vi "Simple Client.vi"() -> ()   [LabVIEW 2023, in "Generated_client.lvlib"]
uses:
  Generated_client.lvlib
  RPC Messages/streamai_signalConfig.ctl
  RPC Messages/streamai_SignalType.ctl
  RPC Messages/streamai_samplingConfig.ctl
  Workers/gRPC Client/gRPC Client.lvclass
panel:
  in  "stop":bool
  out "Waveform Chart":waveform(dbl)(graph)
  in  "Sampling Config":T1={"sample_rate"=1000.0, "num_sample"=100}
  in  "Signal Config":T2={"type"=enum."SIGNAL_SQUARE", "offset"=0.0, "frequency"=5.0, "amplitude"=2.0}
  in  "address":string="localhost:50051"
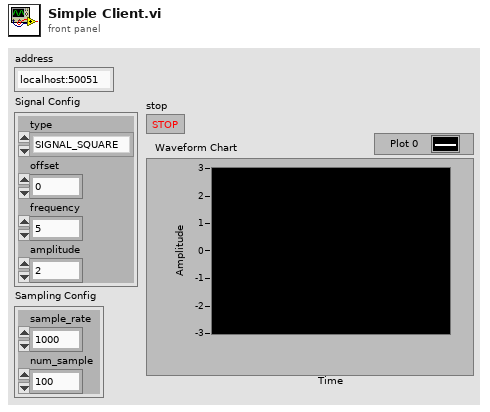
[diagram p1: front panel]
types:
  T1 = typedef "Generated_client.lvlib/streamai_samplingConfig.ctl" = cluster{"sample_rate":dbl, "num_sample":i32}
  T2 = typedef "Generated_client.lvlib/streamai_signalConfig.ctl" = cluster{"type":T3, "offset":dbl, "frequency":dbl, "amplitude":dbl}
  T3 = typedef "Generated_client.lvlib/streamai_SignalType.ctl" = enum32{"SIGNAL_SINE", "SIGNAL_SQUARE"}
  T4 = typedef "grpc-lvsupport-release.lvlib/grpcId.ctl" = u64
  T5 = typedef "Generated_client.lvlib/streamai_waveform.ctl" = cluster{"t0":T6, "delta_t":dbl, "values":dbl[]}
  T6 = typedef "Generated_client.lvlib/google_protobuf_Timestamp.ctl" = cluster{"seconds":i64, "nanos":i32}
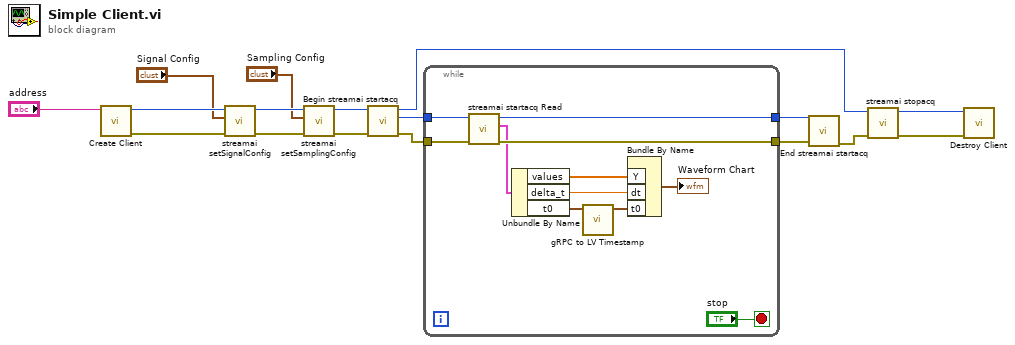
[diagram p0: block diagram]
diagram:
  n1 = call "Create Client.vi"("address"="address") -> ("error out"=w16:errorcluster, "gRPC ID Out"=w17:T4)  [unwired: 9 in]
  n2 = call "streamai setSignalConfig.vi"("error in"=w16, "Request Data"="Signal Config", "gRPC ID"=w17) -> ("error out"=w12:errorcluster, "gRPC ID out"=w13:T4)  [unwired: 6 in, 1 out]
  n3 = call "streamai setSamplingConfig.vi"("error in"=w12, "Request Data"="Sampling Config", "gRPC ID"=w13) -> ("error out"=w9:errorcluster, "gRPC ID out"=w10:T4)  [unwired: 6 in, 1 out]
  n4 = call "Begin streamai startacq.vi"("error in"=w9, "gRPC ID"=w10) -> ("error out"=w8:errorcluster, "Call Id Out"=w4:T4, "gRPC ID out"=w3:T4)  [unwired: 7 in]
  n5 = while {
    tunnel: w4 -> [w28]
    tunnel: w8 -> [w27]
    tunnel: [w26] -> w7
    tunnel: [w25] -> w6
    stop <- "stop" stop-if-true
    n6 = call "streamai startacq Read.vi"("error in"=w27, "Call ID in"=w28) -> ("error out"=w25:errorcluster, "Response Data"=w20:T5, "Call ID"=w26:T4)  [unwired: 6 in, 1 out]
    n7 = Unbundle By Name(w20) -> ("values"=w24:dbl[], "delta_t"=w23:dbl, "t0"=w22:T6)
    n8 = call "gRPC to LV Timestamp.vi"("gRPC Timestamp"=w22) -> ("LV Timestamp"=w21:timestamp)  [unwired: 10 in]
    n9 = Bundle By Name("Y"=w24, "dt"=w23, "t0"=w21) -> (→"Waveform Chart":waveform(dbl))  [unwired: 1 in]
  }
  n10 = call "End streamai startacq.vi"("error in"=w6, "Call ID in"=w7) -> ("error out"=w5:errorcluster)  [unwired: 8 in, 1 out]
  n11 = call "streamai stopacq.vi"("error in"=w5, "gRPC ID"=w3) -> ("error out"=w1:errorcluster, "gRPC ID out"=w2:T4)  [unwired: 7 in, 1 out]
  n12 = call "Destroy Client.vi"("error in"=w1, "gRPC ID"=w2) -> ()  [unwired: 9 in, 1 out]
